vi "35 NEW GPS Interrupt RS232 Read (x64-2018).vi"(2 "Comm Port":refnum<visa-resource-name>) -> (5 "GPS Time Code":string, 6 "CPU Time":dbl format="%#.6f", 7 "VISA Error Out":errorcluster)   [LabVIEW 2017]
uses:
  <vilib>/Instr/_visa.llb/VISA Configure Serial Port (Instr).vi
  NI_Timer.dll
panel:
  out "String":string
  out "Raw String":string
  out "String Length":dbl
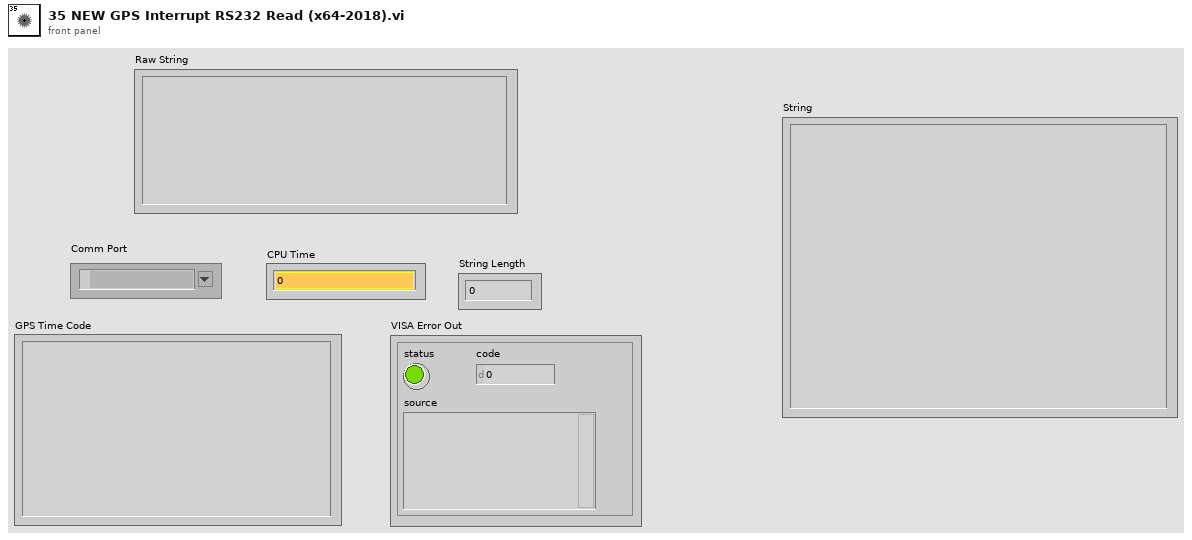
[diagram p1: front panel]
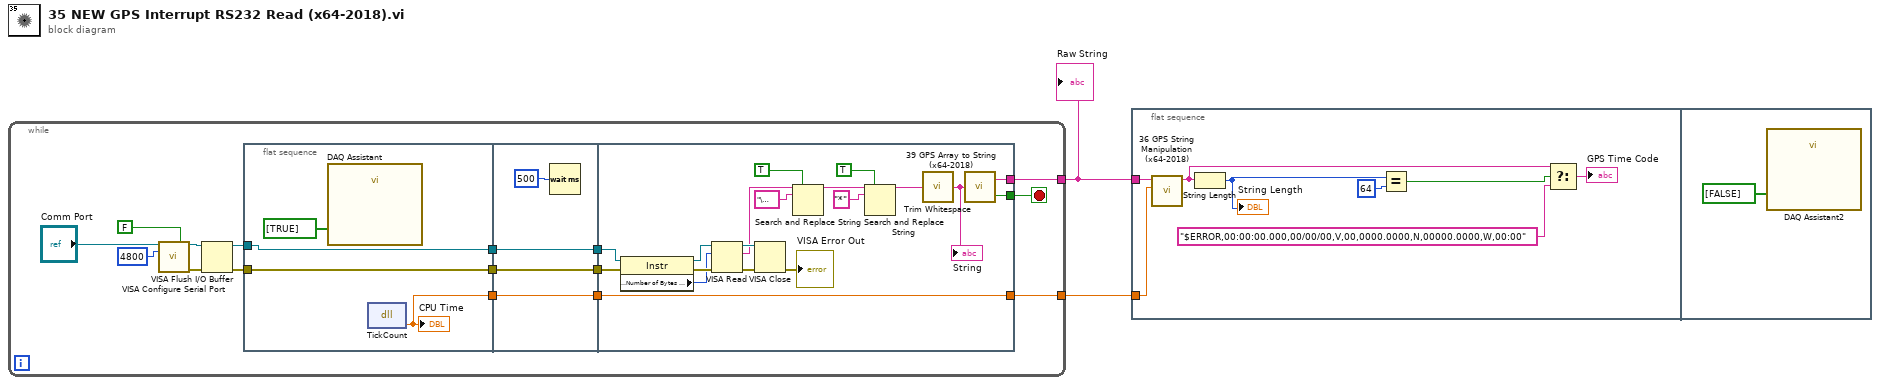
[diagram p0: block diagram]
diagram:
  n1 = while {
    tunnel: [w6] -> w2
    tunnel: [w3] -> w1
    stop <- w7 stop-if-true
    n2 = call-poly "VISA Configure Serial Port"("VISA resource name"="Comm Port", "Enable Termination\nChar (T)"=FALSE ("Enable Termination\nChar (T)"), "baud rate (9600)"=u32 4800) -> ("VISA resource name out"=w12:refnum<visa-resource-name>, "error out"=w11:errorcluster)  [unwired: 11 in]
    n3 = VISA Flush I/O Buffer(VISA resource name=w12, error in (no error)=w11) -> (VISA resource name out=w9:refnum<visa-resource-name>, error out=w10:errorcluster)  [unwired: 1 in]
    n4 = flat-sequence {
      tunnel: [w22] -> w18
      tunnel: w9 -> [w22]
      tunnel: [w21] -> w17
      tunnel: w10 -> [w21]
      tunnel: [w19] -> w4
      tunnel: [w25] -> w16
      tunnel: w18 -> [w25]
      tunnel: [w24] -> w15
      tunnel: w17 -> [w24]
      tunnel: [w23] -> w5
      tunnel: w4 -> [w23]
      tunnel: w16 -> [w45]
      tunnel: w15 -> [w44]
      tunnel: [w30] -> w7
      tunnel: [w29] -> w6
      tunnel: [w28] -> w3
      tunnel: w5 -> [w28]
      frame #0 {
        n5 = call "DAQ Assistant"("data"=bool[] [TRUE]) -> ()  [unwired: 17 in, 2 out]
        n6 = dll-call lib="C:/Users/willie8/Desktop/Research Summer 2K18/Github Upload/Code/Github 64 Bit Upload/NI_Timer.dll" fn="TickCount"() -> ("return type"=w19:dbl)  [unwired: 3 in, 2 out]
        "CPU Time" <- w19
      }
      frame #1 {
        n7 = Wait (ms)(milliseconds to wait=u32 500) -> ()  [unwired: 1 out]
      }
      frame #2 {
        n8 = property class="Instr"(reference=w45, error in=w44) -> (reference out=w43:refnum<visa-resource-name>, error out=w42:errorcluster, "Serial Settings:Number of Bytes at Serial Port"=w39:u32)
        n9 = VISA Read(VISA resource name=w43, byte count=w39, error in (no error)=w42) -> (VISA resource name out=w40:refnum<visa-resource-name>, read buffer=w31:string, error out=w41:errorcluster)  [unwired: 1 out]
        n10 = VISA Close(VISA resource name=w40, error in (no error)=w41) -> (error out=→"VISA Error Out":errorcluster)
        n11 = Search and Replace String(replace all?=TRUE ("replace all? (F)"), input string=w31, search string="\u0000") -> (result string=w34:string)  [unwired: 5 in, 3 out]
        n12 = Search and Replace String(replace all?=TRUE ("replace all? (F)"), input string=w34, search string="*") -> (result string=w33:string)  [unwired: 5 in, 3 out]
        n13 = call <vilib>:"Trim Whitespace.vi"("string"=w33) -> ("trimmed string"=w27:string)  [unwired: 1 in]
        "String" <- w27
        n14 = call "39 GPS Array to String (x64-2018).vi"("Input String"=w27) -> ("Output String"=w29:string, "Code valid?"=w30:bool)
      }
    }
  }
  "Raw String" <- w2
  n15 = flat-sequence {
    tunnel: w2 -> [w47]
    tunnel: w1 -> [w46]
    frame #0 {
      n16 = call "36 GPS String Manipulation (x64-2018).vi"("CPU Time In"=w46, "Input String"=w47) -> ("GPS Time Code"=w53:string)  [unwired: 9 in]
      n17 = String Length(string=w53) -> (length=w52:i32)
      "String Length" <- w52
      n18 = Equal?(x=w52, y=64) -> (x = y?=w50:bool)
      n19 = Select(t=w53, s=w50, f="$ERROR,00:00:00.000,00/00/00,V,00,0000.0000,N,00000.0000,W,00:00") -> (s? t:f=→"GPS Time Code":string)
    }
    frame #1 {
      n20 = call "DAQ Assistant2"("data"=bool[] [FALSE]) -> ()  [unwired: 17 in, 2 out]
    }
  }
